vi "Setup Scope.vi"(0 "instrument handle":refnum<k15>, 5 "channels":string="0", 7 "Scope Parameters":T1={"vertical range"=10.0, "vertical offset"=0.0, "probe attenuation"=1.0, "vertical coupling"=1, "channel enabled"=FALSE, "input impedance"=0, "maximum input frequency"=300000000.0, "min sample rate"=1000000000.0, "reference position"=0.0, "min record length"=50000, "number of records"=1, "enforce realtime"=FALSE} {"min sample rate" format="%#_13g"; "maximum input frequency" format="%#_13p"; "input impedance" items=["1 mega ohm"=0, "50 ohms"=2]; "vertical coupling" items=["AC", "DC", "Ground"]; "probe attenuation" format="%.1f"; "vertical offset" format="%.4f"; "vertical range" format="%#_13g"}, 11 "error in":errorcluster) -> (4 "instrument handle out":refnum<k15>, 15 "error out":errorcluster)   [LabVIEW 2021, in "PMIC Common.lvlib"]
uses:
  PMIC Common.lvlib
  <instrlib>/niScope/Controls/niScope vertical coupling.ctl
  Scope Parameters.ctl
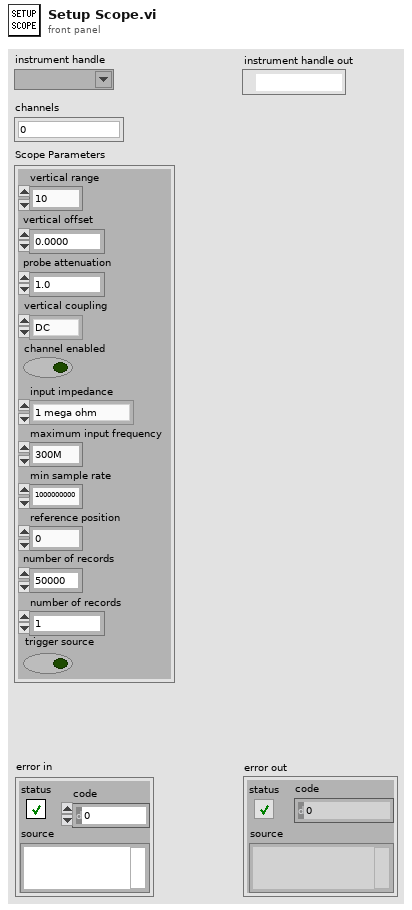
[diagram p1: front panel]
types:
  T1 = typedef "PMIC Common.lvlib/Scope Parameters.ctl" = cluster{"vertical range":dbl, "vertical offset":dbl, "probe attenuation":dbl, "vertical coupling":T2, "channel enabled":bool, "input impedance":u32, "maximum input frequency":dbl, "min sample rate":dbl, "reference position":dbl, "min record length":i32, "number of records":i32, "enforce realtime":bool}
  T2 = typedef "niScope vertical coupling.ctl" = i32
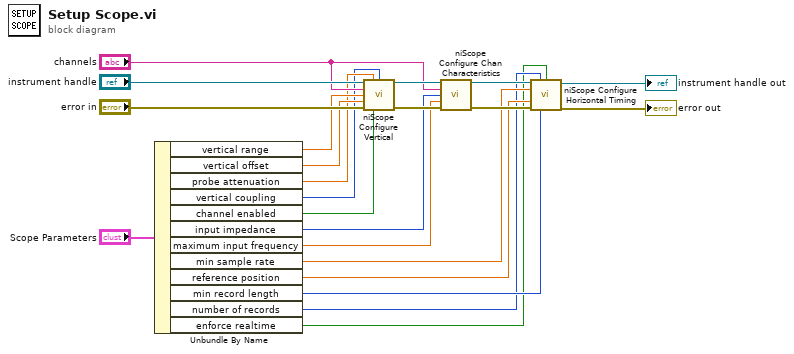
[diagram p0: block diagram]
diagram:
  n1 = Unbundle By Name("Scope Parameters") -> ("vertical range"=w12:dbl, "vertical offset"=w11:dbl, "probe attenuation"=w10:dbl, "vertical coupling"=w9:T2, "channel enabled"=w1:bool, "input impedance"=w14:u32, "maximum input frequency"=w13:dbl, "min sample rate"=w8:dbl, "reference position"=w7:dbl, "min record length"=w6:i32, "number of records"=w5:i32, "enforce realtime"=w4:bool)
  n2 = call <instrlib>:"niScope Configure Vertical.vi"("instrument handle"="instrument handle", "probe attenuation"=w10, "vertical coupling"=w9, "channels"="channels", "vertical range"=w12, "vertical offset"=w11, "error in"="error in", "channel enabled"=w1) -> ("instrument handle out"=w21:refnum<k15>, "error out"=w22:errorcluster)  [unwired: 6 in]
  n3 = call <instrlib>:"niScope Configure Chan Characteristics.vi"("instrument handle"=w21, "channels"="channels", "input impedance"=w14, "maximum input frequency"=w13, "error in"=w22) -> ("instrument handle out"=w19:refnum<k15>, "error out"=w20:errorcluster)  [unwired: 9 in]
  n4 = call <instrlib>:"niScope Configure Horizontal Timing.vi"("instrument handle"=w19, "number of records"=w5, "enforce realtime"=w4, "min sample rate"=w8, "reference position"=w7, "error in"=w20, "min record length"=w6) -> ("instrument handle out"=→"instrument handle out":refnum<k15>, "error out"=→"error out":errorcluster)  [unwired: 7 in]
